vi "MQTT_Connect.vi"(5 "Connect Meta":T5={"QoS"=enum."At most once", "DUP"=FALSE, "Retain"=TRUE, "Keep Alive (sec)"=60}, 6 "Client ID":string="LabVIEW_MQTT_Client", 7 "Connect Flags":T8, 8 "error in (no error)":errorcluster, 9 "Will Info":T6={"Will message"="Last Will", "Will Topic"="Will Topic"}, 10 "User Info":T7={"User Name"="User", "Password"="password"}, 11 "MQTT Broker":cluster{"address (IP)":string, "port":u16}={"address (IP)"="broker.mqttdashboard.com", "port"=1883}) -> (0 "error out":errorcluster, 2 "Connection Status":T1=enum."Connection refused: not authorized", 3 "connection ID out":refnum<k5>)   [LabVIEW 2019, in "MQTT_Functions.lvlib"]
doc: "Connects to an MQTT broker server with required settings. \n\n© 2015 - daq.io, LLC - Peter Adelhardt"
uses:
  MQTT_Functions.lvlib
  Controls/Connect_Flags.ctl
  Controls/QoS.ctl
  Controls/User_Info.ctl
  Controls/Will_Info.ctl
  Controls/DUP_Flag.ctl
  Controls/Retain_Flag.ctl
  Controls/Connection_Return_Codes.ctl
  Controls/Conn_Stat_FGV_Cmds.ctl
  Controls/MessageType.ctl
  Controls/Conn_FGV_Cmds.ctl
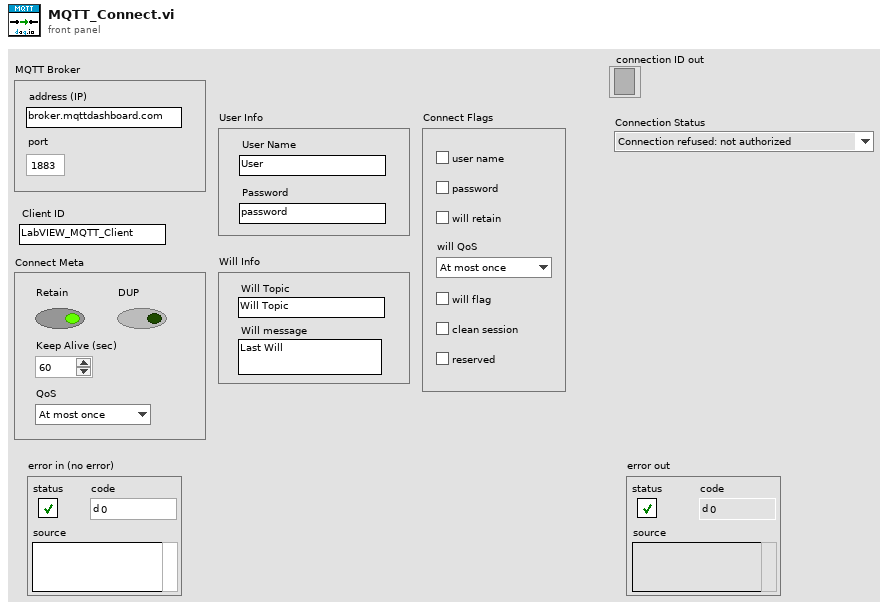
[diagram p1: front panel]
types:
  T1 = typedef "MQTT_Functions.lvlib/Connection_Return_Codes.ctl" = enum16{"Connection accepted", "Connection refused: unacceptable protocol version", "Connection refused: identifier rejected", "Connection refused: Server unavailable", "Connection refused: bad user name or password", "Connection refused: not authorized"}
  T2 = typedef "MQTT_Functions.lvlib/QoS.ctl" = enum8{"At most once", "At least once", "Exactly once", "Reserved"}
  T3 = typedef "MQTT_Functions.lvlib/DUP_Flag.ctl" = bool
  T4 = typedef "MQTT_Functions.lvlib/Retain_Flag.ctl" = bool
  T5 = cluster{"QoS":T2, "DUP":T3, "Retain":T4, "Keep Alive (sec)":u16}
  T6 = typedef "MQTT_Functions.lvlib/Will_Info.ctl" = cluster{"Will message":string, "Will Topic":string}
  T7 = typedef "MQTT_Functions.lvlib/User_Info.ctl" = cluster{"User Name":string, "Password":string}
  T8 = typedef "MQTT_Functions.lvlib/Connect_Flags.ctl" = cluster{"user name":bool, "password":bool, "will retain":bool, "will flag":bool, "clean session":bool, "reserved":bool, "will QoS":T2}
  T9 = typedef "MQTT_Functions.lvlib/Conn_Stat_FGV_Cmds.ctl" = enum16{"Get", "Set"}
  T10 = typedef "MQTT_Functions.lvlib/Conn_FGV_Cmds.ctl" = enum16{"Get", "Set", "Delete"}
  T11 = typedef "MQTT_Functions.lvlib/MessageType.ctl" = enum32{"Reserved", "CONNECT", "CONNACK", "PUBLISH", "PUBACK", "PUBREC", "PUBREL", "PUBCOMP", "SUBSCRIBE", "SUBACK", "UNSUBSCRIBE", "UNSUBACK", "PINGREQ", "PINGRESP", "DISCONNECT", "Reserved2"}
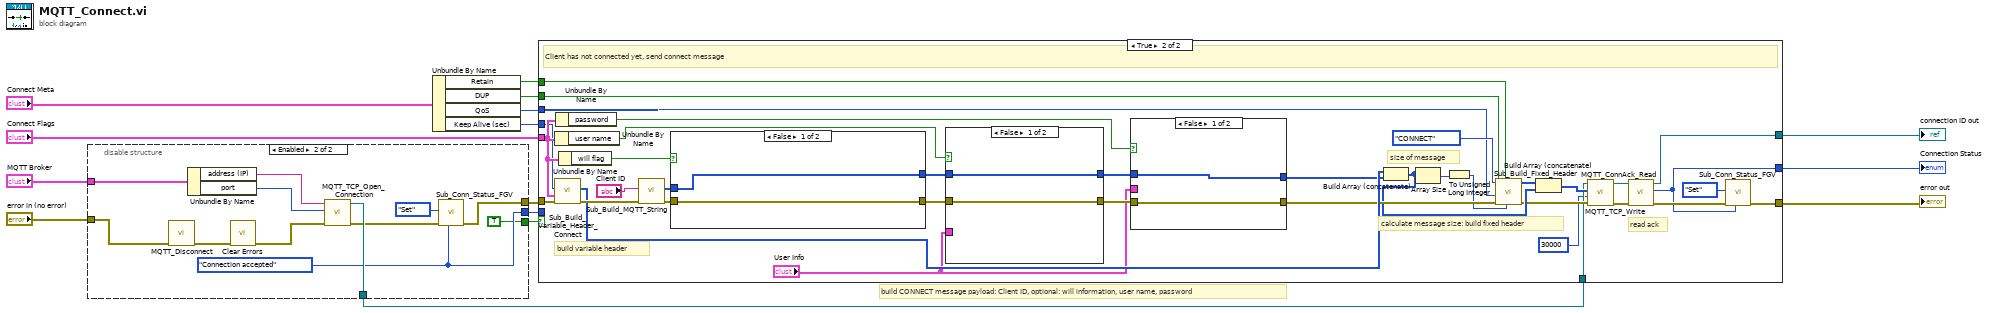
[diagram p0: block diagram]
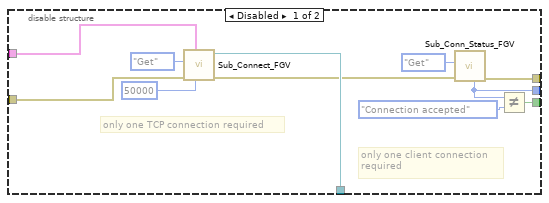
[diagram p2: hidden frame]
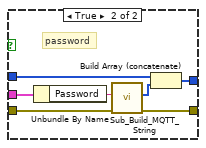
[diagram p4: hidden frame]
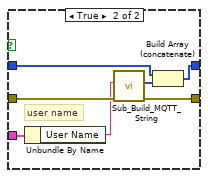
[diagram p5: hidden frame]
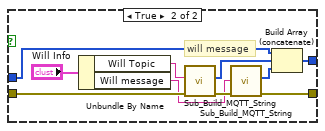
[diagram p6: hidden frame]
diagram:
  # "build CONNECT message payload: Client ID, optional: will information, user name, password"
  n1 = disable-structure shown="Enabled" {
    disable-tunnel: "error in (no error)" -> [w26 w35]
    disable-tunnel: [w25 w34] -> w8
    disable-tunnel: "MQTT Broker" -> [w24 w38]
    disable-tunnel: [w19 TRUE] -> w3
    disable-tunnel: [w18 w29] -> w2
    disable-tunnel: [w17 w28] -> w1
    frame Disabled {
      # "only one client connection\nrequired"
      # "only one TCP connection required"
      n2 = call "Sub_Connect_FGV.vi"("timeout ms (20000)"=50000, "MQTT Broker"=w24, "error in"=w26, "Command"=Conn_FGV_Cmds."Get") -> ("error out"=w21:errorcluster, "MQTT ref out"=w25:refnum<k5>)  [unwired: 6 in]
      n3 = call "Sub_Conn_Status_FGV.vi"("error in"=w21, "Command"=Conn_Stat_FGV_Cmds."Get") -> ("error out"=w18:errorcluster, "Connection Status out"=w17:T1)  [unwired: 8 in]
      n4 = Not Equal?(x=w17, y=Connection_Return_Codes."Connection accepted") -> (x != y?=w19:bool)
    }
    frame Enabled {
      w28 = Connection_Return_Codes."Connection accepted" ("Connection Status in")
      n5 = call "MQTT_Disconnect.vi"("error in (no error)"=w35) -> ("error out"=w33:errorcluster)  [unwired: 10 in]
      n6 = Unbundle By Name(w38) -> ("address (IP)"=w36:string, "port"=w37:u16)
      n7 = call <vilib>:"Clear Errors.vi"("error in (no error)"=w33) -> ("error out"=w32:errorcluster)  [unwired: 5 in, 1 out]
      n8 = call "MQTT_TCP_Open_Connection.vi"("error in (no error)"=w32, "remote port or service name"=w37, "address"=w36) -> ("error out"=w30:errorcluster, "connection ID"=w34:refnum<k5>)  [unwired: 7 in]
      n9 = call "Sub_Conn_Status_FGV.vi"("Connection Status in"=w28, "error in"=w30, "Command"=Conn_Stat_FGV_Cmds."Set") -> ("error out"=w29:errorcluster)  [unwired: 7 in, 1 out]
    }
  }
  n10 = Unbundle By Name("Connect Meta") -> ("Retain"=w13:T4, "DUP"=w12:T3, "QoS"=w11:T2, "Keep Alive (sec)"=w10:u16)
  n11 = case shown="True" w3 {
    tunnel: "Connect Flags" -> [_ w72]
    tunnel: w13 -> [_ w58]
    tunnel: w12 -> [_ w57]
    tunnel: w11 -> [_ w56]
    tunnel: w10 -> [_ w55]
    tunnel: w2 -> [w41 w49]
    tunnel: w8 -> [w39 w48]
    tunnel: [w41 w44] -> w6
    tunnel: [w40 w43] -> w5
    tunnel: [w39 w47] -> w4
    tunnel: w1 -> [w40 _]
    frame False {
      # "client is already connected"
    }
    frame True {
      # "read ack"
      # "calculate message size: build fixed header"
      # "build variable header"
      # "size of message"
      # "Client has not connected yet, send connect message"
      n12 = Unbundle By Name(w72) -> ("user name"=w71:bool)
      n13 = call "Sub_Build_Variable_Header_Connect.vi"("error in (no error)"=w49, "Connect Flags"=w72, "Keep Alive (sec)"=w55) -> ("error out"=w77:errorcluster, "Variable Header"=w68:u8[])  [unwired: 7 in]
      n14 = Unbundle By Name(w72) -> ("password"=w70:bool)
      n15 = Unbundle By Name(w72) -> ("will flag"=w69:bool)
      n16 = call "Sub_Build_MQTT_String.vi"("error in (no error)"=w77, "String to be encoded"="Client ID") -> ("error out"=w73:errorcluster, "UTF8 Byte Array"=w76:u8[])  [unwired: 8 in]
      n17 = case shown="False" w69 {
        tunnel: w76 -> [w98 w106]
        tunnel: [w98 w107] -> w75
        tunnel: w73 -> [w97 w105]
        tunnel: [w97 w102] -> w66
        frame False {
        }
        frame True {
          # "will message"
          n18 = Unbundle By Name("Will Info") -> ("Will Topic"=w100:string, "Will message"=w99:string)
          n19 = call "Sub_Build_MQTT_String.vi"("error in (no error)"=w105, "String to be encoded"=w100) -> ("error out"=w104:errorcluster, "UTF8 Byte Array"=w103:u8[])  [unwired: 8 in]
          n20 = call "Sub_Build_MQTT_String.vi"("error in (no error)"=w104, "String to be encoded"=w99) -> ("error out"=w102:errorcluster, "UTF8 Byte Array"=w108:u8[])  [unwired: 8 in]
          n21 = Build Array (concatenate)(w106, w103, w108) -> (w107:u8[])
        }
      }
      n22 = case shown="False" w71 {
        tunnel: w75 -> [w89 w95]
        tunnel: [w89 w94] -> w74
        tunnel: [w88 w93] -> w67
        tunnel: w66 -> [w88 w92]
        tunnel: "User Info" -> [_ w91]
        frame False {
        }
        frame True {
          # "user name"
          n23 = Unbundle By Name(w91) -> ("User Name"=w90:string)
          n24 = call "Sub_Build_MQTT_String.vi"("error in (no error)"=w92, "String to be encoded"=w90) -> ("error out"=w93:errorcluster, "UTF8 Byte Array"=w96:u8[])  [unwired: 8 in]
          n25 = Build Array (concatenate)(w95, w96) -> (w94:u8[])
        }
      }
      n26 = case shown="False" w70 {
        tunnel: w74 -> [w80 w86]
        tunnel: [w80 w85] -> w64
        tunnel: w67 -> [w79 w84]
        tunnel: [w79 w83] -> w65
        tunnel: "User Info" -> [_ w82]
        frame False {
        }
        frame True {
          # "password"
          n27 = Unbundle By Name(w82) -> ("Password"=w81:string)
          n28 = call "Sub_Build_MQTT_String.vi"("error in (no error)"=w84, "String to be encoded"=w81) -> ("error out"=w83:errorcluster, "UTF8 Byte Array"=w87:u8[])  [unwired: 8 in]
          n29 = Build Array (concatenate)(w86, w87) -> (w85:u8[])
        }
      }
      n30 = Build Array (concatenate)(w68, w64) -> (w63:u8[])
      n31 = Array Size(array=w63) -> (size(s)=w61:i32)
      n32 = To Unsigned Long Integer(number=w61) -> (unsigned 32bit integer=w60:u32)
      n33 = call "Sub_Build_Fixed_Header.vi"("Remaining Length"=w60, "Retain"=w58, "error in (no error)"=w65, "QoS"=w56, "DUP"=w57, "MessageType"=MessageType."CONNECT") -> ("error out"=w53:errorcluster, "Fixed Header"=w62:u8[])  [unwired: 4 in]
      n34 = Build Array (concatenate)(w62, w63) -> (w52:u8[])
      n35 = call "MQTT_TCP_Write.vi"("error in (no error)"=w53, "timeout ms (5000)"=30000, "data in"=w52, "connection ID"=w48) -> ("error out"=w51:errorcluster, "connection ID out"=w50:refnum<k5>)  [unwired: 5 in, 1 out]
      n36 = call "MQTT_ConnAck_Read.vi"("error in (no error)"=w51, "connection ID"=w50) -> ("error out"=w46:errorcluster, "Connection Status"=w43:T1, "connection ID out"=w47:refnum<k5>)  [unwired: 5 in, 2 out]
      n37 = call "Sub_Conn_Status_FGV.vi"("Connection Status in"=w43, "error in"=w46, "Command"=Conn_Stat_FGV_Cmds."Set") -> ("error out"=w44:errorcluster)  [unwired: 7 in, 1 out]
    }
  }
  "error out" <- w6
  "connection ID out" <- w4
  "Connection Status" <- w5
